vi "read-multiple-registers-module.vi"(6 "id":u16, 8 "error in":errorcluster, 9 "regs":u16[](array[numeric]), 10 "number of input registers":u16, 11 "TCP master in":refnum<class "Modbus Master.lvclass">) -> (0 "error out":errorcluster, 2 "Module Cluster":T1, 3 "Modbus master out":refnum<class "Modbus Master.lvclass">)   [LabVIEW 2021]
uses:
  <vilib>/Modbus/master/Modbus Master.lvclass
  General Purpose/BMS.ctl
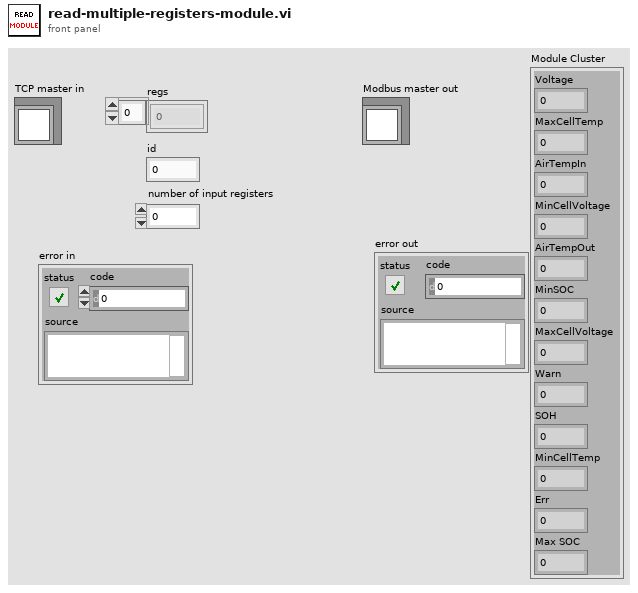
[diagram p1: front panel]
types:
  T1 = cluster{"Voltage":dbl, "MaxCellTemp":dbl, "AirTempIn":dbl, "MinCellVoltage":u16, "AirTempOut":dbl, "MinSOC":u16, "MaxCellVoltage":u16, "Warn":u16, "SOH":u16, "MinCellTemp":dbl, "Err":u16, "Max SOC":u16}
  T2 = typedef "BMS.ctl" = cluster{"rack":cluster{"EoCVoltage":dbl, "MaxChargeCurrent":dbl, "EoDVoltage":dbl, "MaxDischargePower":dbl, "Voltage":dbl, "Current":dbl, "NrOfSRB":u16, "AvgCurrent":dbl, "MaxSOC":u16, "MinSOC":u16, "MaxCellVolt":dbl, "MinCellTemp":dbl, "SOH":u16, "MaxCellTemp":dbl, "AvgCellTemp":dbl, "MinCellVolt":dbl, "MinModVoltage":dbl, "MaxModVoltage":dbl, "Err1":u16, "Warn":u16, "MaxChargePower":dbl, "MaxDischargeCurrent":dbl, "State":string, "ContactorState":string, "OperatingState":string, "Err2":u16}[], "modules":cluster{"Voltage":dbl, "MaxCellTemp":dbl, "AirTempIn":dbl, "MinCellVoltage":u16, "AirTempOut":dbl, "MinSOC":u16, "MaxCellVoltage":u16, "Warn":u16, "SOH":u16, "MinCellTemp":dbl, "Err":u16, "Max SOC":u16}[]}
  T3 = cluster{"Voltage":dbl, "MaxCellTemp":dbl, "AirTempIn":dbl, "MinCellVoltage":u16, "AirTempOut":dbl, "MinSOC":u16, "MaxCellVoltage":u16, "Warn":u16, "SOH":u16, "MinCellTemp":dbl, "Err":u16, "Max SOC":u16}[]
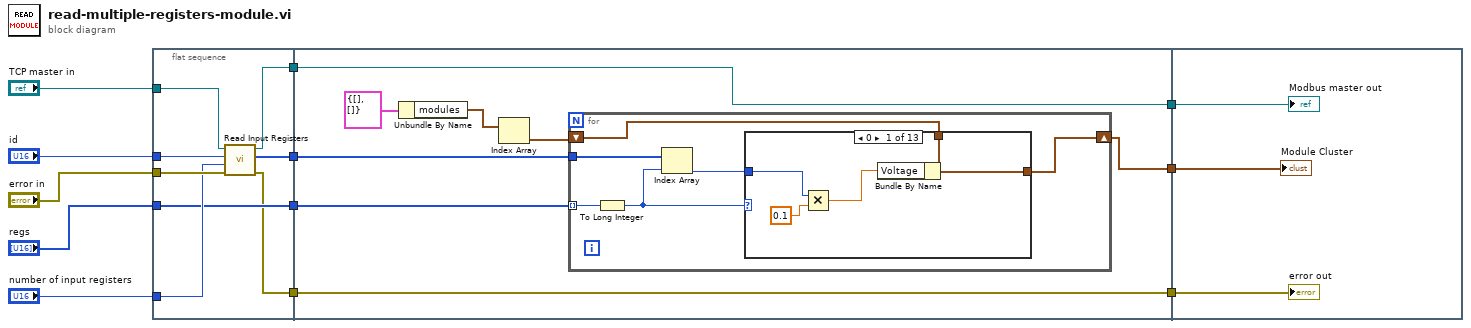
[diagram p0: block diagram]
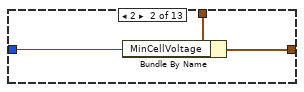
[diagram p2: hidden frame]
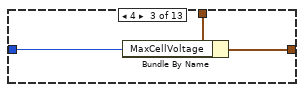
[diagram p3: hidden frame]
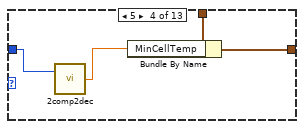
[diagram p4: hidden frame]
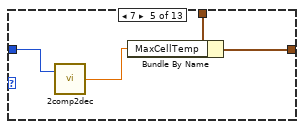
[diagram p5: hidden frame]
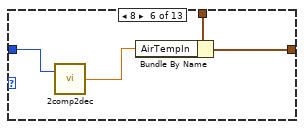
[diagram p6: hidden frame]
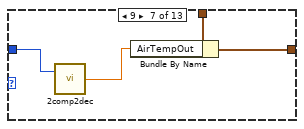
[diagram p7: hidden frame]
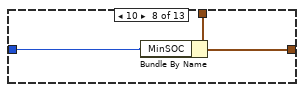
[diagram p8: hidden frame]
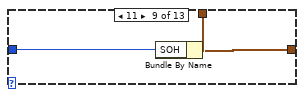
[diagram p9: hidden frame]
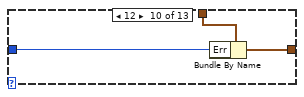
[diagram p10: hidden frame]
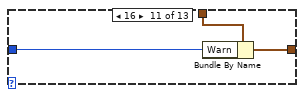
[diagram p11: hidden frame]
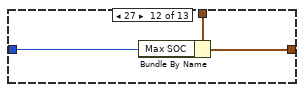
[diagram p12: hidden frame]
diagram:
  n1 = flat-sequence {
    tunnel: "TCP master in" -> [w20]
    tunnel: "id" -> [w19]
    tunnel: "error in" -> [w18]
    tunnel: "number of input registers" -> [w17]
    tunnel: [w16] -> w8
    tunnel: "regs" -> [w16]
    tunnel: [w15] -> w6
    tunnel: [w14] -> w3
    tunnel: [w13] -> w2
    tunnel: w8 -> [w28]
    tunnel: w6 -> [w27]
    tunnel: [w23] -> w5
    tunnel: [w22] -> w4
    tunnel: w3 -> [w22]
    tunnel: w2 -> [w21]
    tunnel: [w21] -> w1
    tunnel: w5 -> [w78]
    tunnel: w4 -> [w80]
    tunnel: w1 -> [w79]
    frame #0 {
      n2 = call-dynamic "Read Input Registers.vi"("error in (no error)"=w18, "number of input registers"=w17, "starting address"=w19, "Modbus master in"=w20) -> ("error out"=w13:errorcluster, "register values"=w15:u16[], "Modbus master out"=w14:refnum<class "Modbus Master.lvclass">)  [unwired: 5 in]
    }
    frame #1 {
      n3 = Unbundle By Name(T2 {"rack"=[], "modules"=[]} ("BMS")) -> ("modules"=w25:T3)
      n4 = Index Array(array=w25) -> (element=w24:T1)  [unwired: 1 in]
      n5 = for {
        tunnel: w28 -> [w34] mode=indexing
        tunnel: w27 -> [w33]
        shift-right: [w29] -> w23
        shift-left: w24 -> [w30]
        n6 = To Long Integer(number=w34) -> (32bit integer=w31:i32)
        n7 = Index Array(array=w33, index=w31) -> (element=w32:u16)
        n8 = case shown="0" w31 {
          tunnel: w32 -> [w37 w40 w43 w47 w51 w55 w59 w62 w65 w68 w71 w74 _]
          tunnel: w30 -> [w39 w42 w45 w49 w53 w57 w61 w64 w67 w70 w73 w76 w77]
          tunnel: [w38 w41 w44 w48 w52 w56 w60 w63 w66 w69 w72 w75 w77] -> w29
          frame 0 {
            n9 = Multiply(x=w37, y=0.1) -> (x*y=w36:dbl)
            n10 = Bundle By Name(cluster=w39, "Voltage"=w36) -> (w38:T1)
          }
          frame 2 {
            n11 = Bundle By Name(cluster=w42, "MinCellVoltage"=w40) -> (w41:T1)
          }
          frame 4 {
            n12 = Bundle By Name(cluster=w45, "MaxCellVoltage"=w43) -> (w44:T1)
          }
          frame 5 {
            n13 = call "2comp2dec.vi"("two' complement"=w47) -> ("decimal"=w46:dbl)  [unwired: 2 in]
            n14 = Bundle By Name(cluster=w49, "MinCellTemp"=w46) -> (w48:T1)
          }
          frame 7 {
            n15 = call "2comp2dec.vi"("two' complement"=w51) -> ("decimal"=w50:dbl)  [unwired: 2 in]
            n16 = Bundle By Name(cluster=w53, "MaxCellTemp"=w50) -> (w52:T1)
          }
          frame 8 {
            n17 = call "2comp2dec.vi"("two' complement"=w55) -> ("decimal"=w54:dbl)  [unwired: 2 in]
            n18 = Bundle By Name(cluster=w57, "AirTempIn"=w54) -> (w56:T1)
          }
          frame 9 {
            n19 = call "2comp2dec.vi"("two' complement"=w59) -> ("decimal"=w58:dbl)  [unwired: 2 in]
            n20 = Bundle By Name(cluster=w61, "AirTempOut"=w58) -> (w60:T1)
          }
          frame 10 {
            n21 = Bundle By Name(cluster=w64, "MinSOC"=w62) -> (w63:T1)
          }
          frame 11 {
            n22 = Bundle By Name(cluster=w67, "SOH"=w65) -> (w66:T1)
          }
          frame 12 {
            n23 = Bundle By Name(cluster=w70, "Err"=w68) -> (w69:T1)
          }
          frame 16 {
            n24 = Bundle By Name(cluster=w73, "Warn"=w71) -> (w72:T1)
          }
          frame 27 {
            n25 = Bundle By Name(cluster=w76, "Max SOC"=w74) -> (w75:T1)
          }
          frame Default {
          }
        }
      }
    }
    frame #2 {
      "error out" <- w79
      "Modbus master out" <- w80
      "Module Cluster" <- w78
    }
  }
